vi "End Preview.vi"(8 "error in (no error)":errorcluster, 10 "Preview":bool, 11 "GUI in":refnum<class "GUI.lvclass">) -> (0 "error out":errorcluster, 3 "GUI out":refnum<class "GUI.lvclass">)   [LabVIEW 2020, in "GUI.lvlib" / "GUI.lvclass"]
uses:
  GUI.lvclass
  GUI.lvclass/GUI.ctl
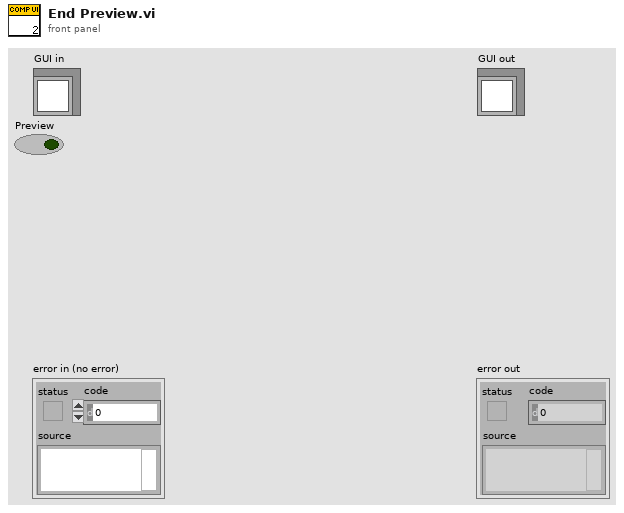
[diagram p1: front panel]
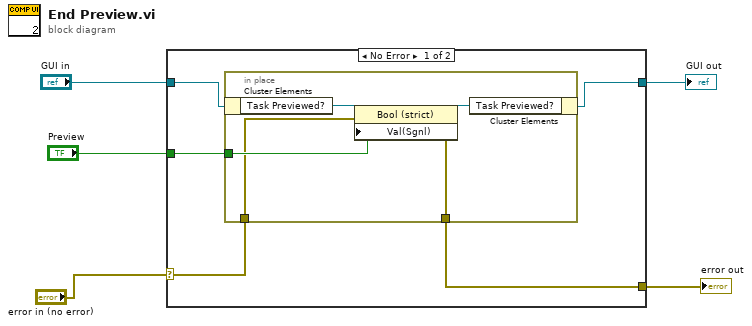
[diagram p0: block diagram]
diagram:
  n1 = case shown="No Error" "error in (no error)" {
    selector: "error in (no error)" -> [w7 w17]
    tunnel: [w6 w17] -> w4
    tunnel: "GUI in" -> [w10 w16]
    tunnel: [w9 w16] -> w2
    tunnel: "Preview" -> [w8 _]
    frame No Error {
      n2 = in-place {
        in-place-border: w8 -> [w13]
        in-place-border: w7 -> [w12]
        in-place-border: [w11] -> w6
        n3 = in-place-cluster #1(w10) -> ("Task Previewed?"=w15:refnum<vi>)
        n4 = property class="Bool (strict)"(reference=w15, error in=w12, "Val(Sgnl)"=w13) -> (reference out=w14:refnum<vi>, error out=w11:errorcluster)
        n5 = in-place-cluster #1("Task Previewed?"=w14) -> (w9:refnum<class "GUI.lvclass">)
      }
    }
    frame Error {
    }
  }
  "error out" <- w4
  "GUI out" <- w2
